vi "Required Font-Scale (As Numeric).vi"(4 "Thickness (Default: 1)":i32=1, 5 "OpenCV Font Face":T1, 8 "error in (no error)":errorcluster, 11 "Required Text Height":u16) -> (0 "error out":errorcluster, 3 "Font Scale":dbl)   [LabVIEW 2020, in "image.lvlib"]
doc: "Compute the Font-Scale for a given Text Height."
uses:
  image.lvlib
  Font Face.ctl
  common/common.lvlib
  common/bin/gartoolkit_32-1.dll
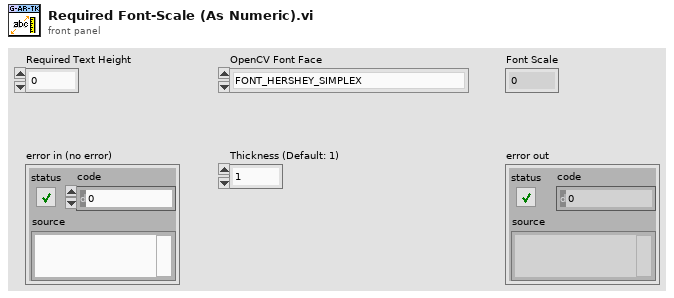
[diagram p1: front panel]
types:
  T1 = typedef "image.lvlib/Font Face.ctl" = enum8{"FONT_HERSHEY_SIMPLEX", "FONT_HERSHEY_PLAIN", "FONT_HERSHEY_DUPLEX", "FONT_HERSHEY_COMPLEX", "FONT_HERSHEY_TRIPLEX", "FONT_HERSHEY_COMPLEX_SMALL", "FONT_HERSHEY_SCRIPT_SIMPLEX", "FONT_HERSHEY_SCRIPT_COMPLEX", "FONT_ITALIC"}
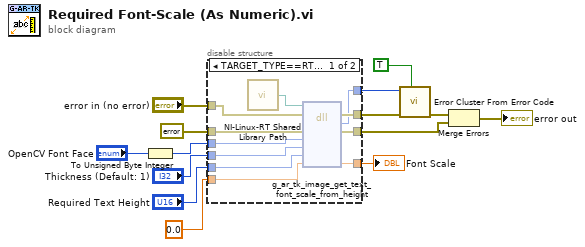
[diagram p0: block diagram]
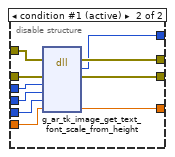
[diagram p2: hidden frame]
diagram:
  n1 = To Unsigned Byte Integer(number="OpenCV Font Face") -> (unsigned 8bit integer=w9:u8)
  n2 = disable-structure shown="TARGET_TYPE==RT&&OS==Linux" {
    disable-tunnel: "error in (no error)" -> [w24 w35]
    disable-tunnel: errorcluster {"status"=FALSE, "code"=0, "source"=""} ("error constant") -> [w23 w34]
    disable-tunnel: w9 -> [w22 w33]
    disable-tunnel: "Thickness (Default: 1)" -> [w21 w32]
    disable-tunnel: "Required Text Height" -> [w20 w31]
    disable-tunnel: 0.0 ("Font Scale") -> [w19 w30]
    disable-tunnel: [w18 w29] -> w5
    disable-tunnel: [w17 w28] -> w4
    disable-tunnel: [w16 w27] -> w3
    disable-tunnel: [w15 w26] -> w2
    frame condition #0 {
      n3 = call "NI-Linux-RT Shared Library Path.vi"() -> ("Path"=w25:path)
      n4 = dll-call lib="?" fn="g_ar_tk_image_get_text_font_scale_from_height"(path in=w25, error in=w24, "error_cluster"=w23, "font_face"=w22, "thickness"=w21, "Required Height"=w20, "Font Scale"=w19) -> (error out=w18:errorcluster, "MgErr"=w17:i32, "error_cluster"=w16:errorcluster, "Font Scale"=w15:dbl)  [unwired: 4 in, 1 out]
    }
    frame condition #1 (active) {
      n5 = dll-call lib="C:/serenial/lib/g-augmented-reality-toolkit/LabVIEW/common/bin/gartoolkit_*-1.*" fn="g_ar_tk_image_get_text_font_scale_from_height"(error in=w35, "error_cluster"=w34, "font_face"=w33, "thickness"=w32, "Required Height"=w31, "Font Scale"=w30) -> (error out=w29:errorcluster, "MgErr"=w28:i32, "error_cluster"=w27:errorcluster, "Font Scale"=w26:dbl)  [unwired: 5 in, 1 out]
    }
  }
  "Font Scale" <- w2
  n6 = call <vilib>:"Error Cluster From Error Code.vi"("show call chain? (False)"=TRUE, "error in (no error)"=w5, "error code (0)"=w4) -> ("error out"=w13:errorcluster)  [unwired: 6 in]
  n7 = Merge Errors(w13, w3) -> (→"error out":errorcluster)
